vi "Sequencer Do.vi"(8 "error in (no error)":errorcluster, 10 "Sequencer in":refnum<class "Sequencer.lvclass">, 11 "Interrupt Sequencer Msg":refnum<class "Flush Sequncer Msg.lvclass">) -> (0 "error out":errorcluster, 2 "Sequencer out":refnum<class "Sequencer.lvclass">)   [LabVIEW 2020, in "Sequencer.lvlib" / "Flush Sequncer Msg.lvclass"]
doc: "The action the Sequencer Msg performs in the Sequencers Recieve Message method.\n\nThis implementation will enqueue itself at the highest priority, send an interrupt and then await completion."
uses:
  Flush Sequncer Msg.lvclass
  C:/Current projects/WS/Framework/Framework/Actors/Sequencer/Sequencer Messages/Sequencer Msg/Sequencer Msg.lvclass
  Sequencer/Sequencer.lvclass
  PPL/HDH.Actor Framework.Core.Actor.lvlibp/1abvi3w/vi.lib/ActorFramework/Message Enqueuer/Message Priority.ctl
  Flush Sequncer Msg.lvclass/Flush Sequncer Msg.ctl
  Sequencer Msg/Sequencer Msg.lvclass/Sequencer Msg.ctl
  Sequencer/Sequencer.lvclass/Sequencer.ctl
  Sequencer Core/Sequencer Core.lvclass/Sequencer Core.ctl
  PPL/HDH.Data.Generic.lvlibp/Synchronization/Notifier/Send.vi
  Sequencer Msg/Sequencer Msg.lvclass
  PPL/HDH.Actor Framework.Core.Actor.lvlibp/1abvi3w/vi.lib/ActorFramework/Message Enqueuer/Message Enqueuer.lvclass
  PPL/HDH.Data.Generic.lvlibp/Synchronization/Notifier/Notifier.lvclass
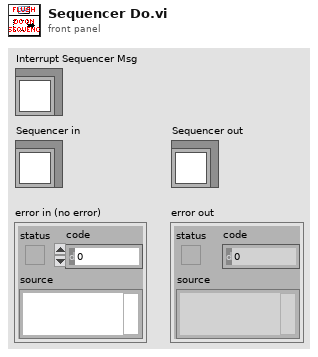
[diagram p1: front panel]
types:
  T1 = typedef "HDH.Actor Framework.Core.Actor.lvlibp/Message Enqueuer.lvclass/Message Priority.ctl" = enum16{"Low", "Normal", "High"}
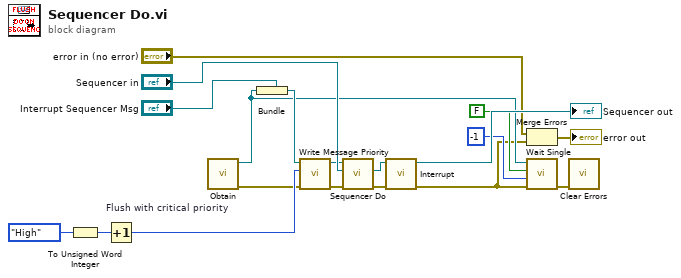
[diagram p0: block diagram]
diagram:
  n1 = To Unsigned Word Integer(number=Message_Priority."High" ("Message Priority")) -> (unsigned 16bit integer=w1:u16)
  n2 = Increment "Flush with critical priority"(x=w1) -> (x+1=w18:u16)
  n3 = call "Obtain.vi"() -> ("error out"=w15:errorcluster, "Notifier out"=w8:refnum<class "Notifier.lvclass">)  [unwired: 9 in, 1 out]
  n4 = Bundle(cluster="Interrupt Sequencer Msg", w8) -> (w16:refnum<class "Flush Sequncer Msg.lvclass">)
  n5 = call "Write Message Priority.vi"("error in (no error)"=w15, "Priority"=w18, "Sequencer Msg in"=w16) -> ("error out"=w12:errorcluster, "Sequencer Msg out"=w13:refnum<class "Flush Sequncer Msg.lvclass">)  [unwired: 7 in]
  n6 = call-parent "Sequencer Do.vi"("error in (no error)"=w12, "Sequencer in"="Sequencer in", "Sequencer Msg"=w13) -> ("error out"=w10:errorcluster, "Sequencer out"=w11:refnum<class "Sequencer.lvclass">)  [unwired: 7 in]
  n7 = call "Interrupt.vi"("error in (no error)"=w10, "Sequencer in"=w11) -> ("error out"=w3:errorcluster, "Sequencer out"=→"Sequencer out":refnum<class "Sequencer.lvclass">)  [unwired: 8 in]
  n8 = Merge Errors("error in (no error)", w3) -> (→"error out":errorcluster)
  n9 = call "Wait Single.vi"("error in (no error)"=w3, "Timeout in ms (-1)"=-1, "Ignore previous (F)"=FALSE, "Notifier in"=w8) -> ("error out"=w5:errorcluster)  [unwired: 4 in, 3 out]
  n10 = call <vilib>:"Clear Errors.vi"("error in (no error)"=w5) -> ()  [unwired: 5 in, 2 out]
